vi "Initialize.vi"(8 "Error In":errorcluster, 11 "Sequencer In":refnum<class "Sequencer.lvclass">) -> (0 "Error Out":errorcluster, 3 "Sequencer Out":refnum<class "Sequencer.lvclass">)   [LabVIEW 2019, in "Sequencer.lvclass"]
uses:
  Sequencer.lvclass
  Process/Process.lvclass
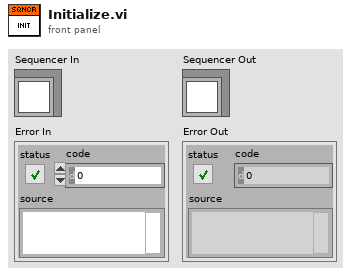
[diagram p1: front panel]
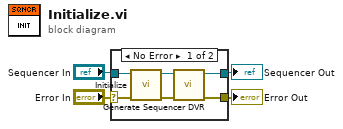
[diagram p0: block diagram]
diagram:
  n1 = case shown="No Error" "Error In" {
    selector: "Error In" -> [w10 w11]
    tunnel: [w6 w11] -> w4
    tunnel: [w5 w12] -> w3
    tunnel: "Sequencer In" -> [w9 w12]
    frame No Error {
      n2 = call-parent "Initialize.vi"("Error In"=w10, "Process In"=w9) -> ("Error Out"=w7:errorcluster, "Process Out"=w8:refnum<class "Sequencer.lvclass">)  [unwired: 8 in]
      n3 = call "Generate Sequencer DVR.vi"("Error In"=w7, "Sequencer In"=w8) -> ("Error Out"=w6:errorcluster, "Sequencer Out"=w5:refnum<class "Sequencer.lvclass">)  [unwired: 8 in]
    }
    frame Error {
    }
  }
  "Sequencer Out" <- w3
  "Error Out" <- w4
